vi "myRIO_BRig_Host_formatData_main.vi"() -> ()   [LabVIEW 2014]
panel:
  in  "error":errorcluster
  in  "input_storagePath":string="C:\\BehaviorRig\\Data\\2016_03_02__Exp1_TM2_run3"
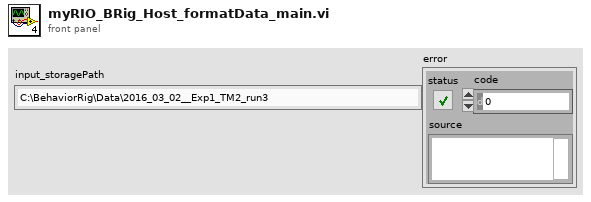
[diagram p1: front panel]
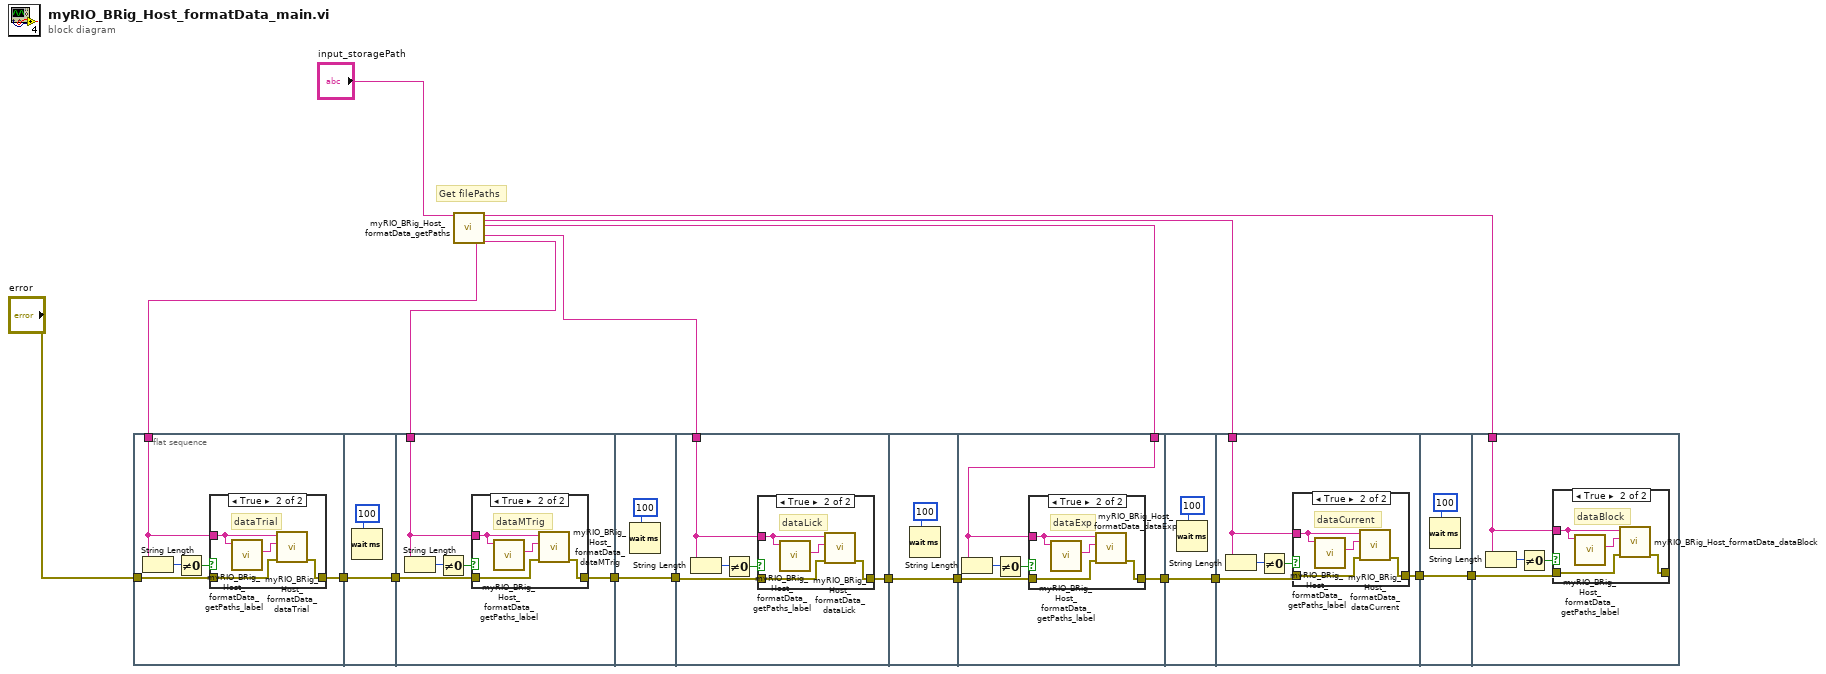
[diagram p0: block diagram]
diagram:
  # "Get filePaths"
  n1 = flat-sequence {
    tunnel: "error" -> [w21]
    tunnel: [w20] -> w2
    tunnel: w1 -> [w19]
    tunnel: [w30] -> w3
    tunnel: w2 -> [w30]
    tunnel: [w33] -> w5
    tunnel: w4 -> [w31]
    tunnel: w3 -> [w32]
    tunnel: [w42] -> w6
    tunnel: w5 -> [w42]
    tunnel: [w45] -> w9
    tunnel: w7 -> [w44]
    tunnel: w6 -> [w43]
    tunnel: [w53] -> w10
    tunnel: w9 -> [w53]
    tunnel: w13 -> [w57]
    tunnel: [w56] -> w17
    tunnel: w10 -> [w55]
    tunnel: w17 -> [w65]
    tunnel: [w65] -> w16
    tunnel: w16 -> [w69]
    tunnel: w11 -> [w68]
    tunnel: [w67] -> w14
    tunnel: [w77] -> w15
    tunnel: w14 -> [w77]
    tunnel: w15 -> [w80]
    tunnel: w12 -> [w79]
    frame #0 {
      n2 = String Length(string=w19) -> (length=w23:i32)
      n3 = Not Equal To 0?(x=w23) -> (x != 0?=w22:bool)
      n4 = case shown="True" w22 {
        tunnel: w19 -> [_ w27]
        tunnel: [w24 w26] -> w20
        tunnel: w21 -> [w24 w25]
        frame False {
        }
        frame True {
          # "dataTrial"
          n5 = call "myRIO_BRig_Host_formatData_getPaths_label.vi"("input_filePath"=w27) -> ("output_filePath_label"=w28:string)  [unwired: 10 in]
          n6 = call "myRIO_BRig_Host_formatData_dataTrial.vi"("input_error"=w25, "input_newPath"=w28, "input_origPath"=w27) -> ("output_error"=w26:errorcluster)  [unwired: 8 in]
        }
      }
    }
    frame #1 {
      n7 = Wait (ms)(milliseconds to wait=u32 100) -> ()  [unwired: 1 out]
    }
    frame #2 {
      n8 = String Length(string=w31) -> (length=w35:i32)
      n9 = Not Equal To 0?(x=w35) -> (x != 0?=w34:bool)
      n10 = case shown="True" w34 {
        tunnel: w31 -> [_ w39]
        tunnel: [w36 w38] -> w33
        tunnel: w32 -> [w36 w37]
        frame False {
        }
        frame True {
          # "dataMTrig"
          n11 = call "myRIO_BRig_Host_formatData_getPaths_label.vi"("input_filePath"=w39) -> ("output_filePath_label"=w40:string)  [unwired: 10 in]
          n12 = call "myRIO_BRig_Host_formatData_dataMTrig.vi"("input_error"=w37, "input_newPath"=w40, "input_origPath"=w39) -> ("output_error"=w38:errorcluster)  [unwired: 8 in]
        }
      }
    }
    frame #3 {
      n13 = Wait (ms)(milliseconds to wait=u32 100) -> ()  [unwired: 1 out]
    }
    frame #4 {
      n14 = String Length(string=w44) -> (length=w47:i32)
      n15 = Not Equal To 0?(x=w47) -> (x != 0?=w46:bool)
      n16 = case shown="True" w46 {
        tunnel: w44 -> [_ w51]
        tunnel: [w48 w50] -> w45
        tunnel: w43 -> [w48 w49]
        frame False {
        }
        frame True {
          # "dataLick"
          n17 = call "myRIO_BRig_Host_formatData_getPaths_label.vi"("input_filePath"=w51) -> ("output_filePath_label"=w52:string)  [unwired: 10 in]
          n18 = call "myRIO_BRig_Host_formatData_dataLick.vi"("input_error"=w49, "input_newPath"=w52, "input_origPath"=w51) -> ("output_error"=w50:errorcluster)  [unwired: 8 in]
        }
      }
    }
    frame #5 {
      n19 = Wait (ms)(milliseconds to wait=u32 100) -> ()  [unwired: 1 out]
    }
    frame #6 {
      n20 = String Length(string=w57) -> (length=w58:i32)
      n21 = Not Equal To 0?(x=w58) -> (x != 0?=w59:bool)
      n22 = case shown="True" w59 {
        tunnel: w57 -> [_ w63]
        tunnel: w55 -> [w60 w62]
        tunnel: [w60 w61] -> w56
        frame False {
        }
        frame True {
          # "dataExp"
          n23 = call "myRIO_BRig_Host_formatData_getPaths_label.vi"("input_filePath"=w63) -> ("output_filePath_label"=w64:string)  [unwired: 10 in]
          n24 = call "myRIO_BRig_Host_formatData_dataExp.vi"("input_error"=w62, "input_newPath"=w64, "input_origPath"=w63) -> ("output_error"=w61:errorcluster)  [unwired: 8 in]
        }
      }
    }
    frame #7 {
      n25 = Wait (ms)(milliseconds to wait=u32 100) -> ()  [unwired: 1 out]
    }
    frame #8 {
      n26 = String Length(string=w68) -> (length=w70:i32)
      n27 = Not Equal To 0?(x=w70) -> (x != 0?=w71:bool)
      n28 = case shown="True" w71 {
        tunnel: w68 -> [_ w75]
        tunnel: w69 -> [w72 w74]
        tunnel: [w72 w73] -> w67
        frame False {
        }
        frame True {
          # "dataCurrent"
          n29 = call "myRIO_BRig_Host_formatData_getPaths_label.vi"("input_filePath"=w75) -> ("output_filePath_label"=w76:string)  [unwired: 10 in]
          n30 = call "myRIO_BRig_Host_formatData_dataCurrent.vi"("input_error"=w74, "input_newPath"=w76, "input_origPath"=w75) -> ("output_error"=w73:errorcluster)  [unwired: 8 in]
        }
      }
    }
    frame #9 {
      n31 = Wait (ms)(milliseconds to wait=u32 100) -> ()  [unwired: 1 out]
    }
    frame #10 {
      n32 = String Length(string=w79) -> (length=w81:i32)
      n33 = Not Equal To 0?(x=w81) -> (x != 0?=w82:bool)
      n34 = case shown="True" w82 {
        tunnel: w79 -> [_ w86]
        tunnel: w80 -> [w83 w85]
        tunnel: [w83 w84] -> _
        frame False {
        }
        frame True {
          # "dataBlock"
          n35 = call "myRIO_BRig_Host_formatData_getPaths_label.vi"("input_filePath"=w86) -> ("output_filePath_label"=w87:string)  [unwired: 10 in]
          n36 = call "myRIO_BRig_Host_formatData_dataBlock.vi"("input_error"=w85, "input_newPath"=w87, "input_origPath"=w86) -> ("output_error"=w84:errorcluster)  [unwired: 8 in]
        }
      }
    }
  }
  n37 = call "myRIO_BRig_Host_formatData_getPaths.vi"("input_storagePath"="input_storagePath") -> ("output_dataTrial"=w1:string, "output_dataBlock"=w12:string, "output_dataCurrent"=w11:string, "output_dataExp"=w13:string, "output_dataLick"=w7:string, "output_dataMTrig"=w4:string)  [unwired: 12 in, 1 out]
